vi "Day 18  - Boiling Boulders.vi"() -> ()   [LabVIEW 2020, in "AoC 2022.lvlib"]
uses:
  AoC 2022.lvlib
  <vilib>/Math Plots/3D Math Plots/3D Scatter/3D Scatter XCtrl/3D Scatter.xctl
  <vilib>/Math Plots/3D Math Plots/3D Scatter/3D Scatter Datatype/Public/Plot Helper (Vector).vi
  <vilib>/Math Plots/3D Math Plots/3D Scatter/3D Scatter Datatype/3D Scatter Datatype.lvclass
panel:
  in  "Lava Droplets 2":i32(listbox)
  in  "Air Pockets Connects to Exterior Srface":i32(listbox)
  in  "Lava Droplets":i32(listbox)
  in  "Trapped Air Pockets":i32(listbox)
  in  "All Locations":i32(listbox)
  out "3D Scatter":refnum<class "3D Plot Datatype.lvclass">[](xcontrol)
  out "Air Pockets S.Area":i32
  out "Puzzle Part-2 Answer 2":i32
  out "Puzzle Part Answer":i32
  out "Puzzle Part-2 Answer":i32
  in  "Puzzle Input":string="2,2,2\n1,2,2\n3,2,2\n2,1,2\n2,3,2\n2,2,1\n2,2,3\n2,2,4\n2,2,6\n1,2,5\n3,2,5\n2,1,5\n2,3,5"
  # "Press Ctrl+M & Enter the Puzzle Input and run the VI"
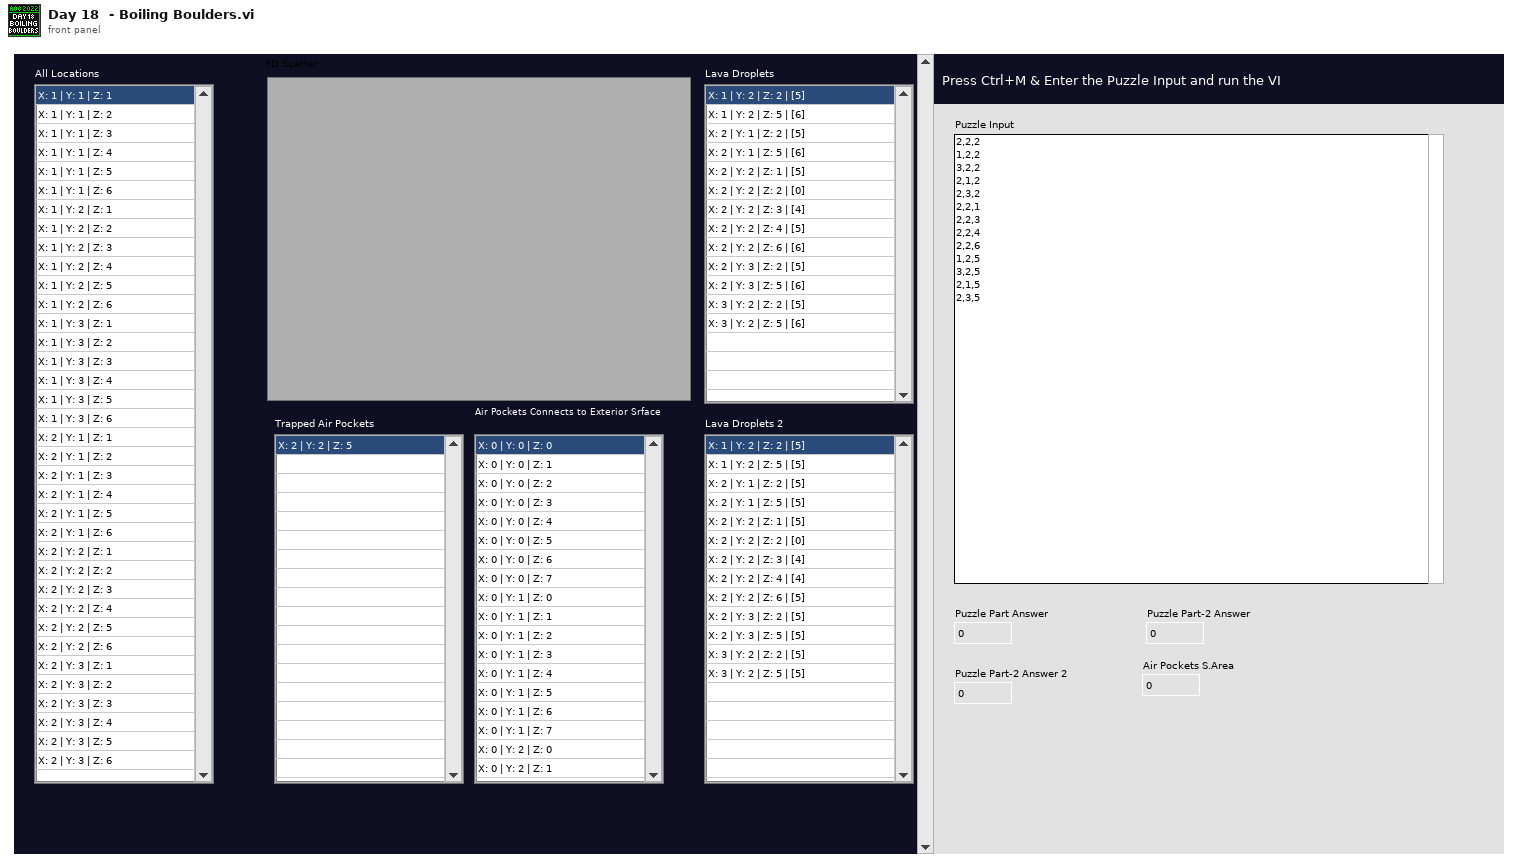
[diagram p1: front panel]
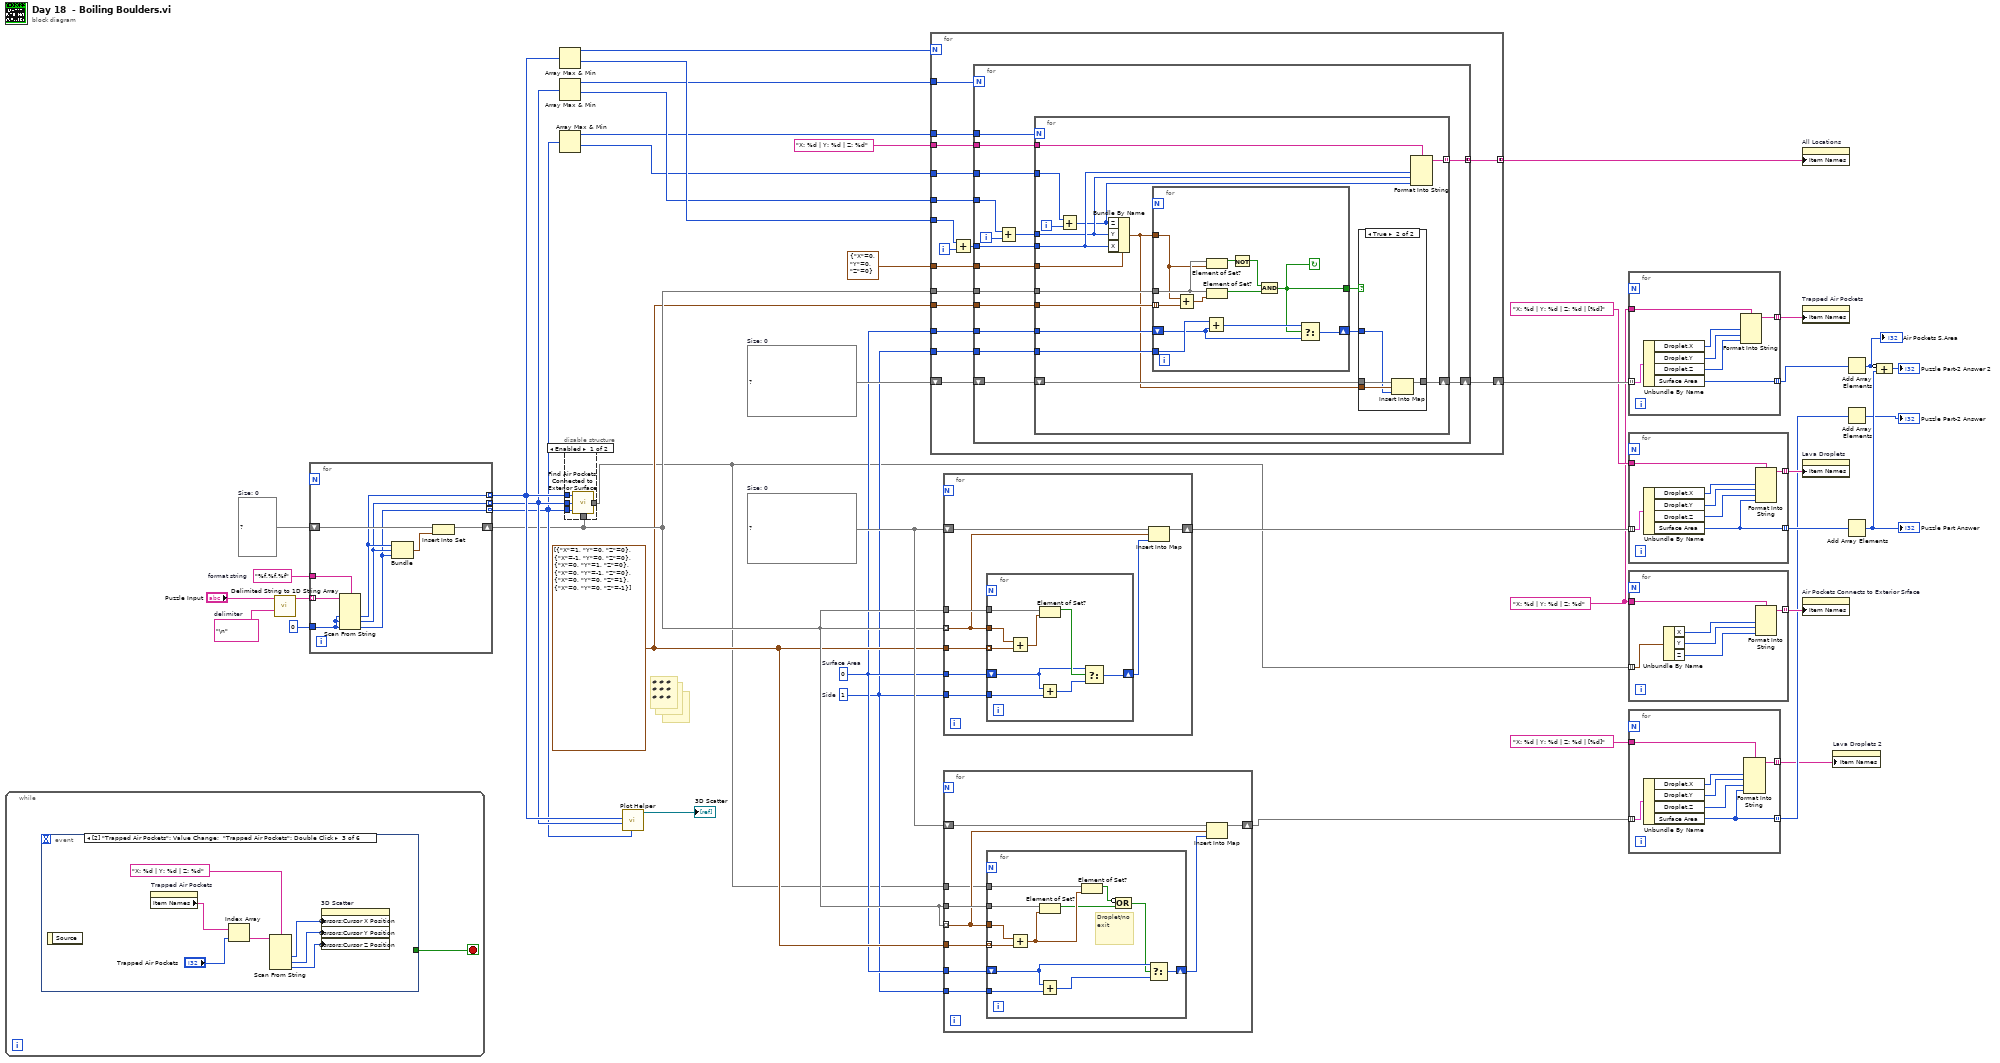
[diagram p0: block diagram]
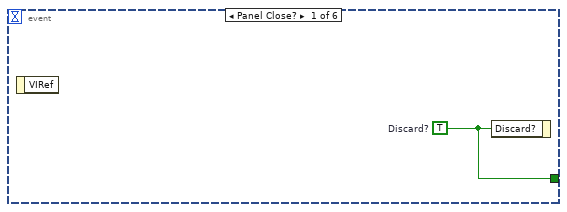
[diagram p3: hidden frame]
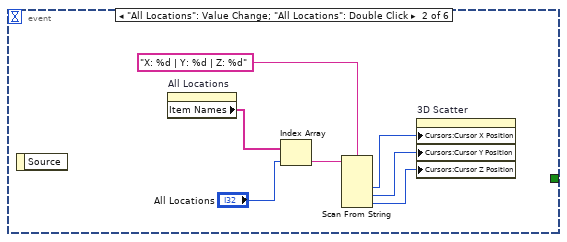
[diagram p4: hidden frame]
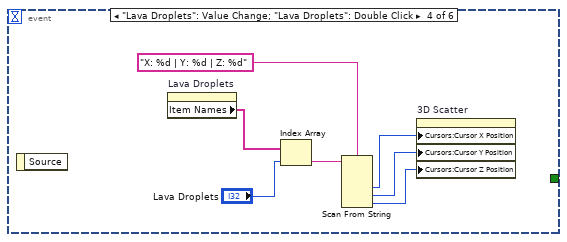
[diagram p5: hidden frame]
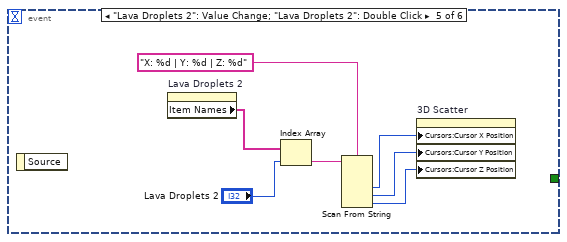
[diagram p6: hidden frame]
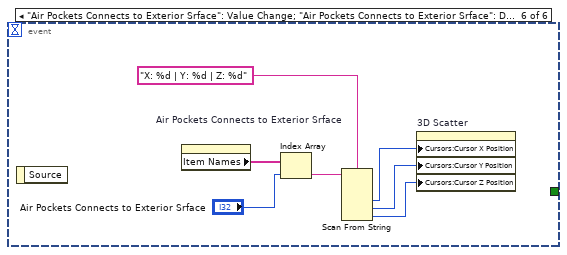
[diagram p7: hidden frame]
diagram:
  w1 = "X: %d | Y: %d | Z: %d"
  w22 = map{cluster{"X":i32, "Y":i32, "Z":i32}, i32} {}  # Size: 0
  w12 = 1  # Side
  w13 = 0  # Surface Area
  w16 = map{cluster{"X":i32, "Y":i32, "Z":i32}, i32} {}  # Size: 0
  w14 = cluster{"X":i32, "Y":i32, "Z":i32}[] [{"X"=1, "Y"=0, "Z"=0}, {"X"=-1, "Y"=0, "Z"=0}, {"X"=0, "Y"=1, "Z"=0}, {"X"=0, "Y"=-1, "Z"=0}, {"X"=0, "Y"=0, "Z"=1}, {"X"=0, "Y"=0, "Z"=-1}]
  w38 = set{cluster{"X":i32, "Y":i32, "Z":i32}} {}  # Size: 0
  w40 = "%f,%f,%f"  # format string
  w43 = "\n"  # delimiter
  # "# # #\n# # #\n# # #"
  # "# # #\n# # #\n# # #"
  # "# # #\n# # #\n# # #"
  n1 = while {
    stop <- w44 stop-if-true
    n2 = event shown="[2] \"Trapped Air Pockets\": Value Change;  \"Trapped Air Pockets\": Double Click" {
      selector: _ -> [_ _ _ _ _ _]
      dyn-events: _ -> [_ _ _ _ _ _]
      timeout: _ -> [_ _ _ _ _ _]
      tunnel: [w45 _ _ _ _ _] -> w44
      event Panel Close? {
        w45 = TRUE  # Discard?
        n3 = event-data() -> ()  [unwired: 1 in, 1 out]
        n4 = event-data("Discard?"=w45) -> ()  [unwired: 1 in, 1 out]
      }
      event "All Locations": Value Change; "All Locations": Double Click {
        n5 = event-data() -> ()  [unwired: 1 in, 1 out]
        n6 = property on="All Locations" class="LstBox (strict)"() -> ("Item Names"=w52:string[])  [unwired: 2 in, 2 out]
        n7 = Index Array(array=w52, index="All Locations") -> (element=w51:string)
        n8 = Scan From String(format string="X: %d | Y: %d | Z: %d", input string=w51) -> (output 1=w49:i32, output 2=w48:i32, output 3=w47:i32)  [unwired: 5 in, 3 out]
        n9 = property on="3D Scatter" class="3D Scatter (strict)"("Cursors:Cursor X Position"=w49, "Cursors:Cursor Y Position"=w48, "Cursors:Cursor Z Position"=w47) -> ()  [unwired: 2 in, 2 out]
      }
      event "Trapped Air Pockets": Value Change; "Trapped Air Pockets": Double Click {
        n10 = event-data() -> ()  [unwired: 1 in, 1 out]
        n11 = property on="Trapped Air Pockets" class="LstBox (strict)"() -> ("Item Names"=w59:string[])  [unwired: 2 in, 2 out]
        n12 = Index Array(array=w59, index="Trapped Air Pockets") -> (element=w58:string)
        n13 = Scan From String(format string="X: %d | Y: %d | Z: %d", input string=w58) -> (output 1=w56:i32, output 2=w55:i32, output 3=w54:i32)  [unwired: 5 in, 3 out]
        n14 = property on="3D Scatter" class="3D Scatter (strict)"("Cursors:Cursor X Position"=w56, "Cursors:Cursor Y Position"=w55, "Cursors:Cursor Z Position"=w54) -> ()  [unwired: 2 in, 2 out]
      }
      event "Lava Droplets": Value Change; "Lava Droplets": Double Click {
        n15 = event-data() -> ()  [unwired: 1 in, 1 out]
        n16 = property on="Lava Droplets" class="LstBox (strict)"() -> ("Item Names"=w66:string[])  [unwired: 2 in, 2 out]
        n17 = Index Array(array=w66, index="Lava Droplets") -> (element=w65:string)
        n18 = Scan From String(format string="X: %d | Y: %d | Z: %d", input string=w65) -> (output 1=w63:i32, output 2=w62:i32, output 3=w61:i32)  [unwired: 5 in, 3 out]
        n19 = property on="3D Scatter" class="3D Scatter (strict)"("Cursors:Cursor X Position"=w63, "Cursors:Cursor Y Position"=w62, "Cursors:Cursor Z Position"=w61) -> ()  [unwired: 2 in, 2 out]
      }
      event "Lava Droplets 2": Value Change; "Lava Droplets 2": Double Click {
        n20 = event-data() -> ()  [unwired: 1 in, 1 out]
        n21 = property on="Lava Droplets 2" class="LstBox (strict)"() -> ("Item Names"=w73:string[])  [unwired: 2 in, 2 out]
        n22 = Index Array(array=w73, index="Lava Droplets 2") -> (element=w72:string)
        n23 = Scan From String(format string="X: %d | Y: %d | Z: %d", input string=w72) -> (output 1=w70:i32, output 2=w69:i32, output 3=w68:i32)  [unwired: 5 in, 3 out]
        n24 = property on="3D Scatter" class="3D Scatter (strict)"("Cursors:Cursor X Position"=w70, "Cursors:Cursor Y Position"=w69, "Cursors:Cursor Z Position"=w68) -> ()  [unwired: 2 in, 2 out]
      }
      event "Air Pockets Connects to Exterior Srface": Value Change; "Air Pockets Connects to Exterior Srface": Double Click {
        n25 = event-data() -> ()  [unwired: 1 in, 1 out]
        n26 = property on="Air Pockets Connects to Exterior Srface" class="LstBox (strict)"() -> ("Item Names"=w75:string[])  [unwired: 2 in, 2 out]
        n27 = Index Array(array=w75, index="Air Pockets Connects to Exterior Srface") -> (element=w80:string)
        n28 = Scan From String(format string="X: %d | Y: %d | Z: %d", input string=w80) -> (output 1=w78:i32, output 2=w77:i32, output 3=w76:i32)  [unwired: 5 in, 3 out]
        n29 = property on="3D Scatter" class="3D Scatter (strict)"("Cursors:Cursor X Position"=w78, "Cursors:Cursor Y Position"=w77, "Cursors:Cursor Z Position"=w76) -> ()  [unwired: 2 in, 2 out]
      }
    }
  }
  n30 = call <vilib>:"Delimited String to 1D String Array.vi"("delimiter"=w43, "delimited string"="Puzzle Input") -> ("string array"=w41:string[])  [unwired: 9 in]
  n31 = for {
    tunnel: w41 -> [w89] mode=indexing
    tunnel: w40 -> [w88]
    tunnel: 0 -> [w87]
    shift-right: [w84] -> w15
    shift-left: w38 -> [w86]
    tunnel: [w83] -> w21 mode=indexing
    tunnel: [w82] -> w20 mode=indexing
    tunnel: [w81] -> w19 mode=indexing
    n32 = Scan From String(format string=w88, input string=w89, default 1=w87, default 2=w87, default 3=w87) -> (output 1=w83:i32, output 2=w82:i32, output 3=w81:i32)  [unwired: 2 in, 3 out]
    n33 = Bundle(w83, w82, w81) -> (w85:cluster{i32, i32, i32})  [unwired: 1 in]
    n34 = Insert Into Set(10:w85, 11:w86) -> (3:w84:set{cluster{"X":i32, "Y":i32, "Z":i32}})  [unwired: 1 out]
  }
  n35 = Array Max & Min(array=w21) -> (max value=w35:i32, min value=w34:i32)  [unwired: 2 out]
  n36 = Array Max & Min(array=w20) -> (max value=w33:i32, min value=w32:i32)  [unwired: 2 out]
  n37 = Array Max & Min(array=w19) -> (max value=w31:i32, min value=w30:i32)  [unwired: 2 out]
  n38 = disable-structure shown="Enabled" {
    disable-tunnel: w21 -> [w94 _]
    disable-tunnel: w20 -> [w93 _]
    disable-tunnel: w19 -> [w92 _]
    disable-tunnel: w15 -> [w91 _]
    disable-tunnel: [w90 _] -> w11
    frame Enabled {
      n39 = call "Find Air Pockets Connected to Exterior Surface.vi"("Lava Droplets"=w91, "Z"=w92, "Y"=w93, "X"=w94) -> ("Air Pockets Connected to Exterior Surface"=w90:set{cluster{"X":i32, "Y":i32, "Z":i32}})
    }
    frame Disabled {
    }
  }
  n40 = call-poly <vilib>:"Plot Helper.vi"("z vector"=w19, "y vector"=w20, "x vector"=w21) -> ("3D Plot lvclass Array out"=→"3D Scatter":refnum<class "3D Plot Datatype.lvclass">[])  [unwired: 3 in, 5 out]
  n41 = for {
    N: w35 -> [_]
    tunnel: w15 -> [w101]
    tunnel: w34 -> [w109]
    tunnel: w33 -> [w108]
    tunnel: w32 -> [w107]
    tunnel: w31 -> [w106]
    tunnel: w30 -> [w105]
    tunnel: cluster{"X":i32, "Y":i32, "Z":i32} {"X"=0, "Y"=0, "Z"=0} -> [w104]
    tunnel: w14 -> [w100]
    tunnel: w13 -> [w99]
    tunnel: w12 -> [w98]
    shift-right: [w97] -> w28
    shift-left: w22 -> [w102]
    tunnel: "X: %d | Y: %d | Z: %d" -> [w96]
    tunnel: [w95] -> w25 mode=concatenating
    i -> [w110]
    n42 = Add(x=w109, y=w110) -> (x+y=w103:i32)
    n43 = for {
      N: w108 -> [_]
      tunnel: w107 -> [w125]
      tunnel: w106 -> [w123]
      tunnel: w105 -> [w122]
      tunnel: w104 -> [w121]
      tunnel: w103 -> [w120]
      tunnel: w101 -> [w117]
      tunnel: w100 -> [w116]
      tunnel: w99 -> [w115]
      tunnel: w98 -> [w114]
      shift-right: [w113] -> w97
      shift-left: w102 -> [w118]
      tunnel: w96 -> [w112]
      tunnel: [w111] -> w95 mode=concatenating
      i -> [w124]
      n44 = Add(x=w125, y=w124) -> (x+y=w119:i32)
      n45 = for {
        N: w123 -> [_]
        tunnel: w122 -> [w141]
        tunnel: w121 -> [w140]
        tunnel: w120 -> [w130]
        tunnel: w119 -> [w129]
        tunnel: w117 -> [w139]
        tunnel: w116 -> [w138]
        tunnel: w115 -> [w137]
        tunnel: w114 -> [w136]
        shift-right: [w134] -> w113
        shift-left: w118 -> [w135]
        tunnel: w112 -> [w127]
        tunnel: [w126] -> w111 mode=indexing
        i -> [w142]
        n46 = Add(x=w141, y=w142) -> (x+y=w128:i32)
        n47 = Bundle By Name(cluster=w140, "Z"=w128, "Y"=w129, "X"=w130) -> (w133:cluster{"X":i32, "Y":i32, "Z":i32})
        n48 = for {
          tunnel: w133 -> [w152]
          tunnel: w139 -> [w153]
          tunnel: w138 -> [w159] mode=indexing
          shift-right: [w154] -> w132
          shift-left: w137 -> [w155]
          tunnel: w136 -> [w157]
          tunnel: [w148] -> w131
          stop <- w148 continue-if-true
          n49 = Add(x=w152, y=w159) -> (x+y=w158:cluster{"X":i32, "Y":i32, "Z":i32})
          n50 = Add(x=w157, y=w155) -> (x+y=w156:i32)
          n51 = Element of Set?(10:w152, 11:w153) -> (3:w151:bool)
          n52 = Element of Set?(10:w158, 11:w153) -> (3:w149:bool)
          n53 = Not(x=w151) -> (.not. x?=w150:bool)
          n54 = And(x=w150, y=w149) -> (x .and. y?=w148:bool)
          n55 = Select(t=w156, s=w148, f=w155) -> (s? t:f=w154:i32)
        }
        n56 = case shown="True" w131 {
          tunnel: w135 -> [w143 w147]
          tunnel: [w143 w146] -> w134
          tunnel: w133 -> [_ w145]
          tunnel: w132 -> [_ w144]
          frame False {
          }
          frame True {
            n57 = Insert Into Map(map in=w147, key=w145, value=w144) -> (map out=w146:map{cluster{"X":i32, "Y":i32, "Z":i32}, i32})  [unwired: 2 out]
          }
        }
        n58 = Format Into String(format string=w127, w130, w129, w128) -> (resulting string=w126:string)  [unwired: 2 in, 1 out]
      }
    }
  }
  n59 = for {
    tunnel: w15 -> [w163] mode=indexing
    tunnel: w15 -> [w167]
    tunnel: w14 -> [w166]
    shift-right: [w164] -> w37
    shift-left: w16 -> [w165]
    tunnel: w13 -> [w162]
    tunnel: w12 -> [w160]
    n60 = for {
      tunnel: w163 -> [w175]
      tunnel: w167 -> [w176]
      tunnel: w166 -> [w174] mode=indexing
      shift-right: [w168] -> w161
      shift-left: w162 -> [w169]
      tunnel: w160 -> [w172]
      n61 = Add(x=w175, y=w174) -> (x+y=w173:cluster{"X":i32, "Y":i32, "Z":i32})
      n62 = Add(x=w169, y=w172) -> (x+y=w171:i32)
      n63 = Element of Set?(10:w173, 11:w176) -> (3:w170:bool)
      n64 = Select(t=w169, s=w170, f=w171) -> (s? t:f=w168:i32)
    }
    n65 = Insert Into Map(map in=w165, key=w163, value=w161) -> (map out=w164:map{cluster{"X":i32, "Y":i32, "Z":i32}, i32})  [unwired: 2 out]
  }
  n66 = for {
    tunnel: w15 -> [w181] mode=indexing
    tunnel: w15 -> [w185]
    tunnel: w14 -> [w184]
    shift-right: [w182] -> w10
    shift-left: w16 -> [w183]
    tunnel: w13 -> [w180]
    tunnel: w12 -> [w178]
    tunnel: w11 -> [w177]
    n67 = for {
      tunnel: w181 -> [w196]
      tunnel: w185 -> [w197]
      tunnel: w184 -> [w195] mode=indexing
      shift-right: [w191] -> w179
      shift-left: w180 -> [w192]
      tunnel: w178 -> [w194]
      tunnel: w177 -> [w190]
      # "Droplet/no exit"
      n68 = Add(x=w196, y=w195) -> (x+y=w189:cluster{"X":i32, "Y":i32, "Z":i32})
      n69 = Add(x=w192, y=w194) -> (x+y=w193:i32)
      n70 = Element of Set?(10:w189, 11:w197) -> (3:w188:bool)
      n71 = Element of Set?(10:w189, 11:w190) -> (3:w187:bool)
      n72 = Compound Arithmetic op=OR(invert w187, w188) -> (w186:bool)
      n73 = Select(t=w192, s=w186, f=w193) -> (s? t:f=w191:i32)
    }
    n74 = Insert Into Map(map in=w183, key=w181, value=w179) -> (map out=w182:map{cluster{"X":i32, "Y":i32, "Z":i32}, i32})  [unwired: 2 out]
  }
  n75 = for {
    tunnel: w28 -> [w204] mode=indexing
    tunnel: [w198] -> w4 mode=indexing
    tunnel: w1 -> [w200]
    tunnel: [w199] -> w24 mode=indexing
    n76 = Unbundle By Name(w204) -> ("Droplet.X"=w203:i32, "Droplet.Y"=w202:i32, "Droplet.Z"=w201:i32, "Surface Area"=w198:i32)
    n77 = Format Into String(format string=w200, w203, w202, w201) -> (resulting string=w199:string)  [unwired: 2 in, 1 out]
  }
  n78 = for {
    tunnel: w37 -> [w208] mode=indexing
    tunnel: [w205] -> w36 mode=indexing
    tunnel: "X: %d | Y: %d | Z: %d | [%d]" -> [w207]
    tunnel: [w206] -> w23 mode=indexing
    n79 = Unbundle By Name(w208) -> ("Droplet.X"=w209:i32, "Droplet.Y"=w210:i32, "Droplet.Z"=w211:i32, "Surface Area"=w205:i32)
    n80 = Format Into String(format string=w207, w209, w210, w211, w205) -> (resulting string=w206:string)  [unwired: 2 in, 1 out]
  }
  n81 = for {
    tunnel: w11 -> [w214] mode=indexing
    tunnel: w1 -> [w213]
    tunnel: [w212] -> w17 mode=indexing
    n82 = Unbundle By Name(w214) -> ("X"=w215:i32, "Y"=w216:i32, "Z"=w217:i32)
    n83 = Format Into String(format string=w213, w215, w216, w217) -> (resulting string=w212:string)  [unwired: 2 in, 1 out]
  }
  n84 = for {
    tunnel: w10 -> [w224] mode=indexing
    tunnel: [w218] -> w9 mode=indexing
    tunnel: "X: %d | Y: %d | Z: %d | [%d]" -> [w223]
    tunnel: [w219] -> w7 mode=indexing
    n85 = Unbundle By Name(w224) -> ("Droplet.X"=w222:i32, "Droplet.Y"=w221:i32, "Droplet.Z"=w220:i32, "Surface Area"=w218:i32)
    n86 = Format Into String(format string=w223, w222, w221, w220, w218) -> (resulting string=w219:string)  [unwired: 2 in, 1 out]
  }
  n87 = property on="All Locations" class="LstBox (strict)"("Item Names"=w25) -> ()  [unwired: 2 in, 2 out]
  n88 = property on="Trapped Air Pockets" class="LstBox (strict)"("Item Names"=w24) -> ()  [unwired: 2 in, 2 out]
  n89 = property on="Lava Droplets" class="LstBox (strict)"("Item Names"=w23) -> ()  [unwired: 2 in, 2 out]
  n90 = property on="Air Pockets Connects to Exterior Srface" class="LstBox (strict)"("Item Names"=w17) -> ()  [unwired: 2 in, 2 out]
  n91 = property on="Lava Droplets 2" class="LstBox (strict)"("Item Names"=w7) -> ()  [unwired: 2 in, 2 out]
  n92 = Add Array Elements(numeric array=w4) -> (sum=w5:i32)
  "Air Pockets S.Area" <- w5
  n93 = Add Array Elements(numeric array=w9) -> (sum=→"Puzzle Part-2 Answer":i32)
  n94 = Add Array Elements(numeric array=w36) -> (sum=w3:i32)
  "Puzzle Part Answer" <- w3
  n95 = Compound Arithmetic op=ADD(invert w5, w3) -> (→"Puzzle Part-2 Answer 2":i32)
